vi "telnet operation.vi"() -> ()   [LabVIEW 2014]
uses:
  <vilib>/addons/internet/NI_InternetTK_Core_VIs.lvlib
panel:
  out "data out 3":string
  out "data out 2":string
  out "data out":string
  in  "address":string="192.68.1.2"
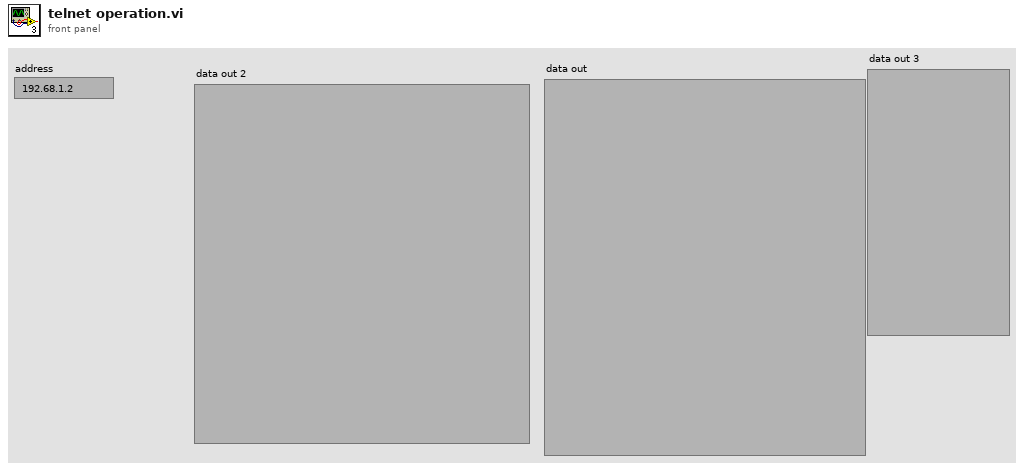
[diagram p1: front panel]
types:
  T1 = typedef "Telnet Session.ctl" = refnum<k1>
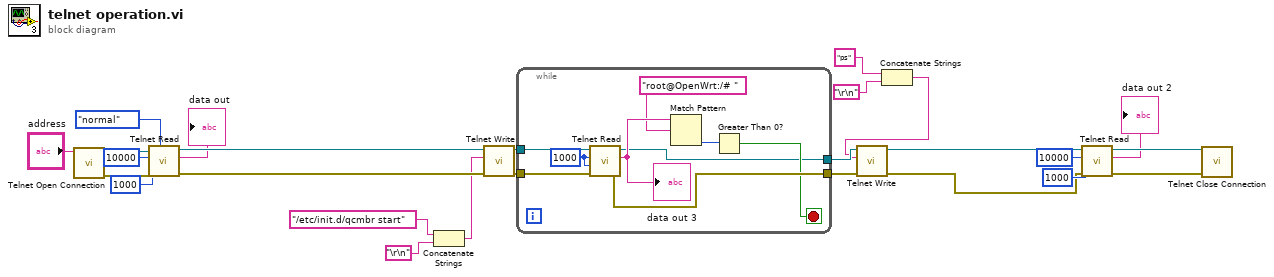
[diagram p0: block diagram]
diagram:
  n1 = call <vilib>:"Telnet Open Connection.vi"("address"="address") -> ("error out"=w25:errorcluster, "telnet connection"=w26:T1)  [unwired: 9 in]
  n2 = call <vilib>:"Telnet Read.vi"("read mode (normal)"=enum16{"normal", "line", "buffered"}."normal", "error in (no error)"=w25, "timeout ms (25000)"=1000, "bytes to read"=10000, "telnet connection"=w26) -> ("error out"=w24:errorcluster, "data out"=→"data out":string, "telnet connection out"=w22:T1)  [unwired: 2 in]
  n3 = Concatenate Strings("/etc/init.d/qcmbr start" ("data in"), "\r\n") -> (w4:string)
  n4 = call <vilib>:"Telnet Write.vi"("error in (no error)"=w24, "data in"=w4, "telnet connection"=w22) -> ("error out"=w10:errorcluster, "telnet connection out"=w11:T1)  [unwired: 4 in, 1 out]
  n5 = while {
    tunnel: w11 -> [w35]
    tunnel: [w27] -> w7
    tunnel: w10 -> [w34]
    tunnel: [w33] -> w9
    stop <- w29 stop-if-true
    w28 = 1000 ("bytes to read")
    n6 = call <vilib>:"Telnet Read.vi"("error in (no error)"=w34, "timeout ms (25000)"=w28, "bytes to read"=w28, "telnet connection"=w35) -> ("error out"=w33:errorcluster, "data out"=w32:string, "telnet connection out"=w27:T1)  [unwired: 3 in]
    "data out 3" <- w32
    n7 = Match Pattern(string=w32, regular expression="root@OpenWrt:/# ") -> (offset past match=w30:i32)  [unwired: 1 in, 3 out]
    n8 = Greater Than 0?(x=w30) -> (x > 0?=w29:bool)
  }
  n9 = Concatenate Strings("ps" ("data in"), "\r\n") -> (w1:string)
  n10 = call <vilib>:"Telnet Write.vi"("error in (no error)"=w9, "data in"=w1, "telnet connection"=w7) -> ("error out"=w8:errorcluster, "telnet connection out"=w14:T1)  [unwired: 4 in, 1 out]
  n11 = call <vilib>:"Telnet Read.vi"("error in (no error)"=w8, "timeout ms (25000)"=1000, "bytes to read"=10000, "telnet connection"=w14) -> ("error out"=w23:errorcluster, "data out"=→"data out 2":string, "telnet connection out"=w21:T1)  [unwired: 3 in]
  n12 = call <vilib>:"Telnet Close Connection.vi"("error in (no error)"=w23, "telnet connection"=w21) -> ()  [unwired: 8 in, 2 out]
